vi "Assign Pixel to Wing Sector (FPGA).vi"(4 "End of Data?":bool, 6 "Valid Data?":bool, 7 "Pixel Intensity In":u8, 8 "Right Wing?":bool, 9 "Sector Parameters":T1, 10 "Pixel Y":u16, 11 "Pixel X":u16) -> (0 "Y":u16, 1 "Pixel Intensity Out":u8, 2 "sector #":u8, 3 "output valid":bool, 5 "X":u16)   [LabVIEW 2013]
uses:
  Sector Parameter Cluster.ctl
  <vilib>/rvi/FXPMathLib/FxpRectToPolar/XNode/nifxpmath_RectToPolar.xnode
  <vilib>/rvi/FXPMathLib/FxpSub/XNode/nifxpmath_Sub.xnode
  <vilib>/rvi/FXPMathLib/sim/FxpSim.dll
  <vilib>/rvi/FXPMathLib/FxpAdd/XNode/nifxpmath_Add.xnode
  <vilib>/rvi/FXPMathLib/FxpDiv/XNode/nifxpmath_Div.xnode
  <vilib>/rvi/FXPMathLib/FxpRectToPolar/simVIs/DllFxpRectToPolarTemp_sub.vi
  <vilib>/rvi/FXPMathLib/FxpRectToPolar/subVIs/nifxpmath_RectToPolar_SimConfig.ctl
  <vilib>/ptbypt/NI_PtbyPt.lvlib
  <vilib>/rvi/FXPMathLib/FxpDiv/simVIs/DllFxpDivTemp_sub.vi
  <vilib>/rvi/FXPMathLib/FxpDiv/subVIs/nifxpmath_Div_SimConfig.ctl
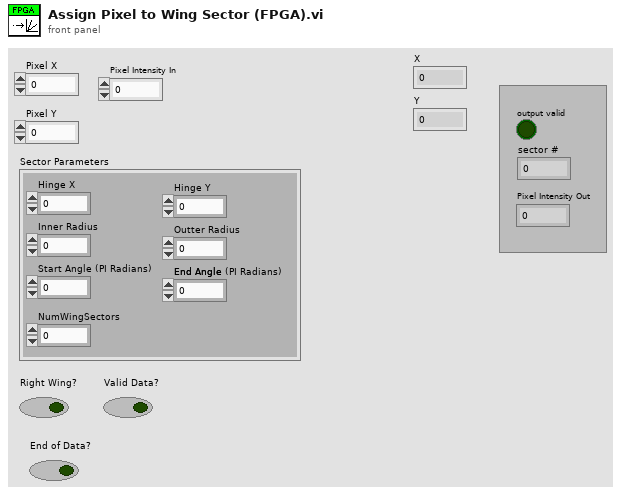
[diagram p1: front panel]
types:
  T1 = typedef "Sector Parameter Cluster.ctl" = cluster{"Start Angle":fxp<+/-,17,2>, "End Angle":fxp<+/-,17,2>, "Inner Radius":u16, "Outter Radius":u16, "Hinge X":u16, "Hinge Y":u16, "NumWingSectors":u8}
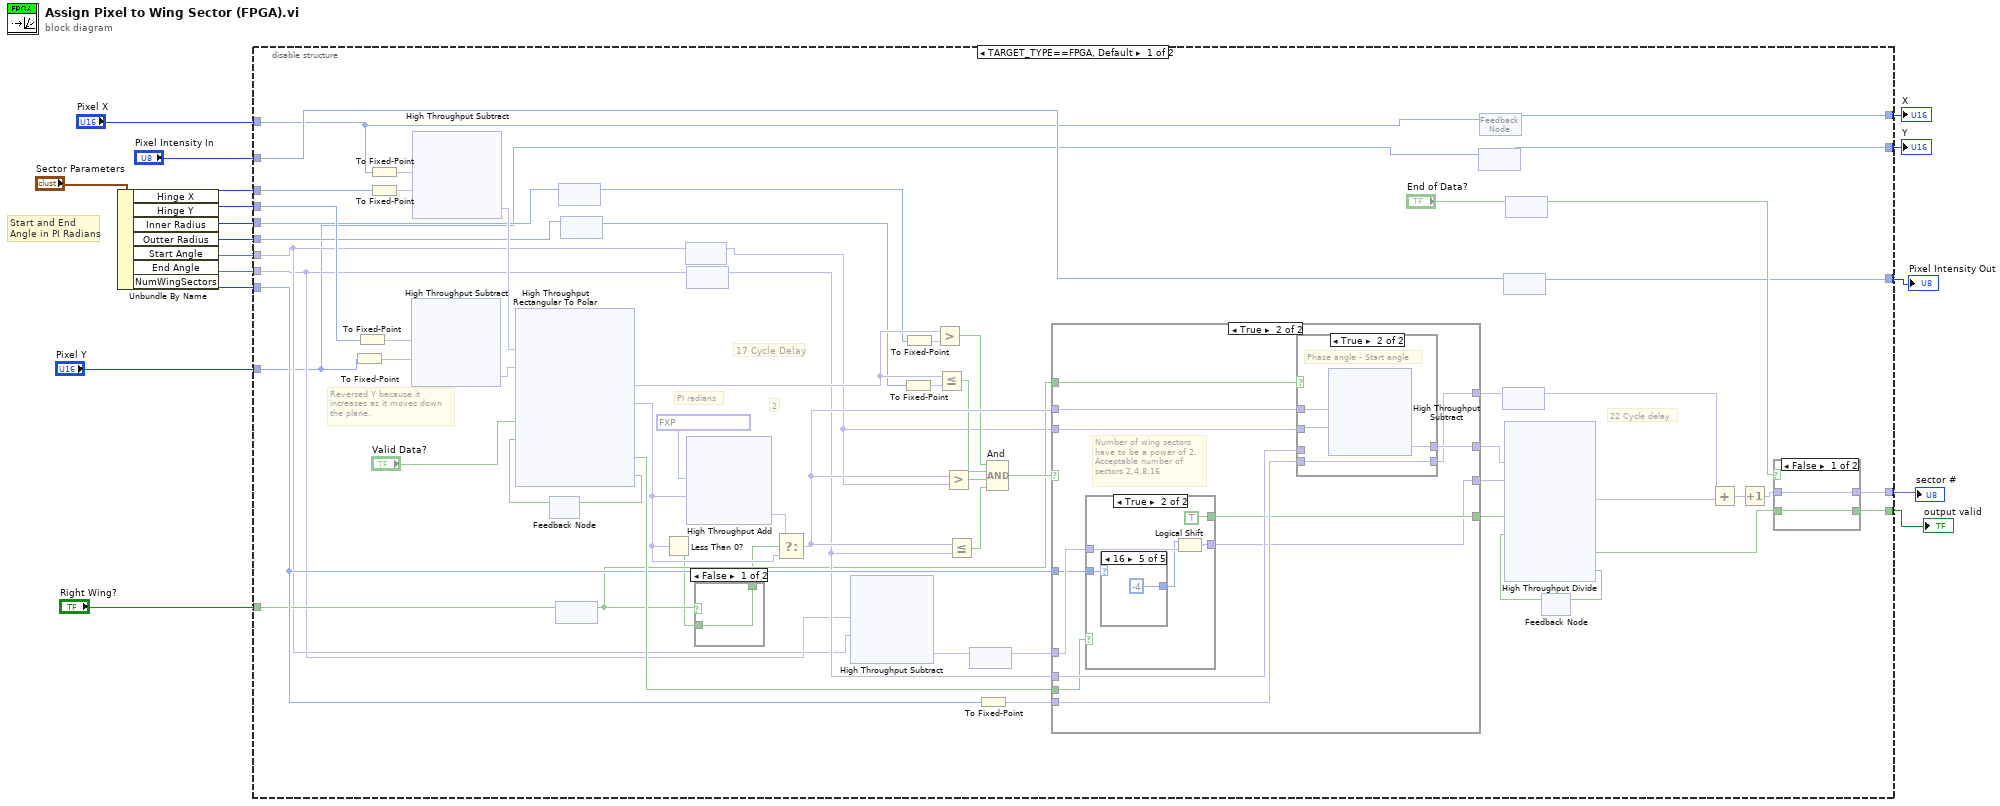
[diagram p0: block diagram]
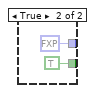
[diagram p2: hidden frame]
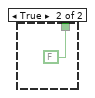
[diagram p3: hidden frame]
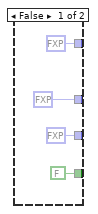
[diagram p4: hidden frame]
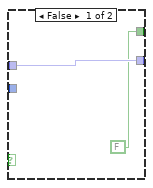
[diagram p5: hidden frame]
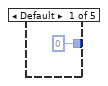
[diagram p6: hidden frame]
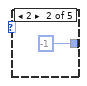
[diagram p7: hidden frame]
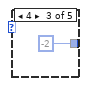
[diagram p8: hidden frame]
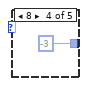
[diagram p9: hidden frame]
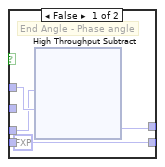
[diagram p10: hidden frame]
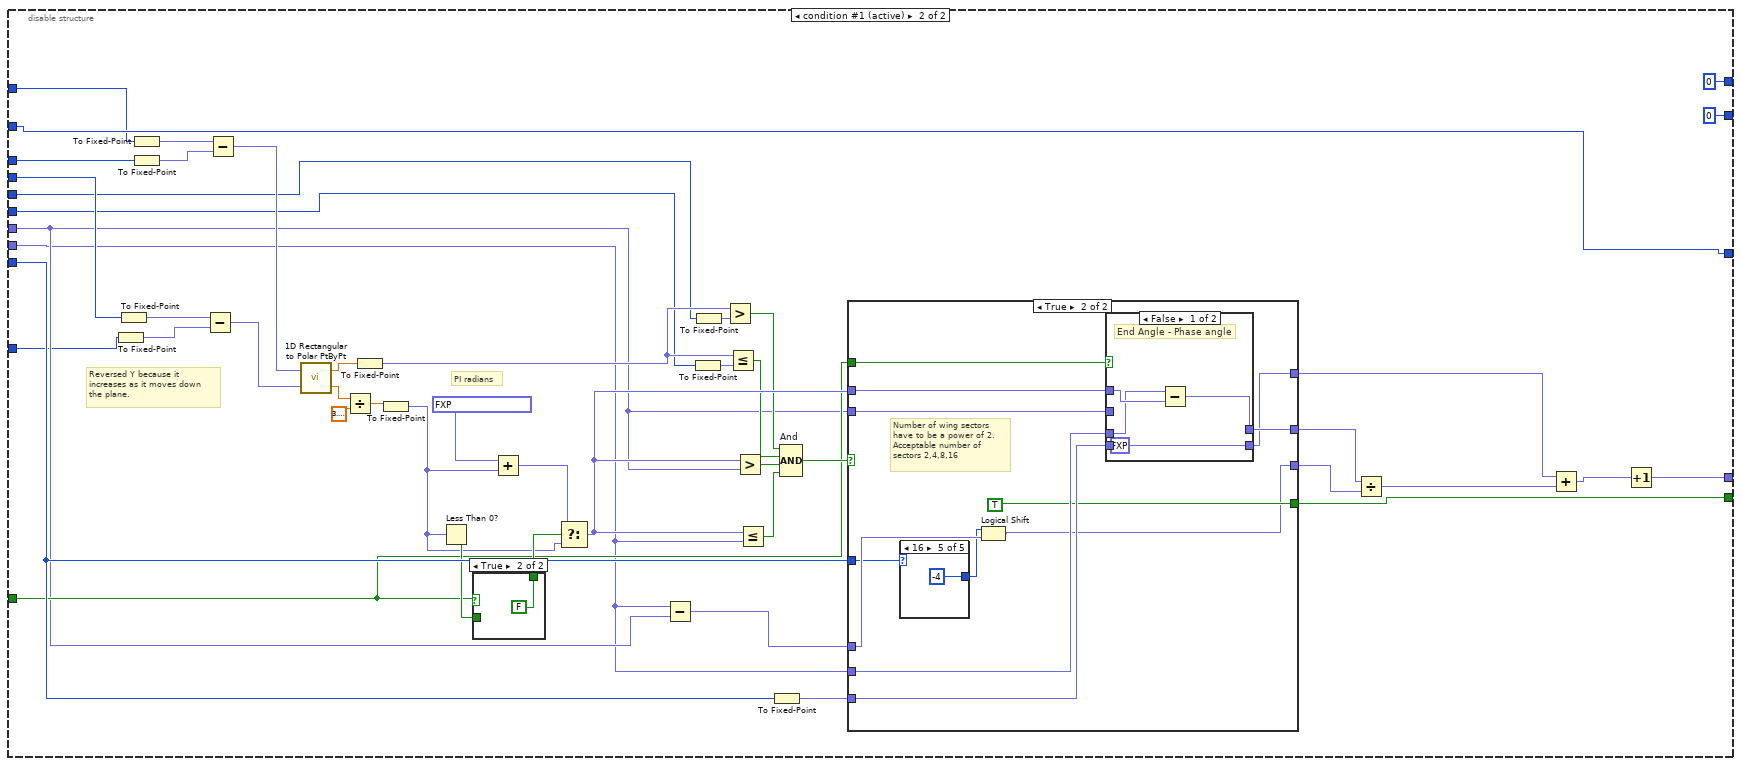
[diagram p11: hidden frame]
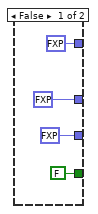
[diagram p13: hidden frame]
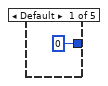
[diagram p14: hidden frame]
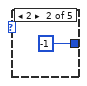
[diagram p15: hidden frame]
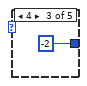
[diagram p16: hidden frame]
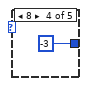
[diagram p17: hidden frame]
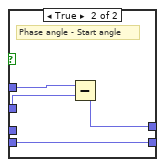
[diagram p18: hidden frame]
diagram:
  # "Start and End\nAngle in PI Radians"
  n1 = Unbundle By Name("Sector Parameters") -> ("Hinge X"=w15:u16, "Hinge Y"=w17:u16, "Inner Radius"=w13:u16, "Outter Radius"=w12:u16, "Start Angle"=w10:fxp<+/-,17,2>, "End Angle"=w9:fxp<+/-,17,2>, "NumWingSectors"=w16:u8)
  n2 = disable-structure shown="TARGET_TYPE==FPGA, Default" {
    disable-tunnel: w17 -> [w64 w224]
    disable-tunnel: w16 -> [w50 w216]
    disable-tunnel: w15 -> [w49 w215]
    disable-tunnel: w13 -> [w48 w204]
    disable-tunnel: w12 -> [w46 w203]
    disable-tunnel: "Right Wing?" -> [w40 w205]
    disable-tunnel: w10 -> [w37 w202]
    disable-tunnel: w9 -> [w35 w201]
    disable-tunnel: [w29 w192] -> w8
    disable-tunnel: [w27 w196] -> w7
    disable-tunnel: "Pixel X" -> [w21 w198]
    disable-tunnel: "Pixel Y" -> [w19 w197]
    disable-tunnel: [w25 w199] -> w4
    disable-tunnel: "Pixel Intensity In" -> [w22 w199]
    disable-tunnel: [w20 u16 0 ("Pixel X")] -> w2
    disable-tunnel: [w18 u16 0 ("Pixel Y")] -> w1
    frame condition #0 {
      # "17 Cycle Delay"
      # "Reversed Y because it\nincreases as it moves down\nthe plane."
      # "PI radians"
      # "22 Cycle delay"
      # "2"
      n3 = To Fixed-Point(number=w19) -> (fixed-point=w54:fxp<+,11,11>)  [unwired: 1 in]
      n4 = To Fixed-Point(number=w64) -> (fixed-point=w55:fxp<+,11,11>)  [unwired: 1 in]
      n5 = To Fixed-Point(number=w21) -> (fixed-point=w53:fxp<+,11,11>)  [unwired: 1 in]
      n6 = To Fixed-Point(number=w49) -> (fixed-point=w52:fxp<+,11,11>)  [unwired: 1 in]
      n7 = xnode "High Throughput Subtract"("x"=w55, "y"=w54) -> ("x-y"=w63:fxp<+/-,12,12>)
      n8 = xnode "High Throughput Subtract"("x"=w53, "y"=w52) -> ("x-y"=w62:fxp<+/-,12,12>)
      n9 = feedback #1() -> (w69:bool)  [unwired: 1 in]
      n10 = xnode "High Throughput Rectangular To Polar"("x"=w62, "y"=w63, "input valid"="Valid Data?", "ready for output (T)"=w69) -> ("magnitude"=w77:fxp<+,12,12>, "phase (pi)"=w74:fxp<+/-,16,2>, "output valid"=w51:bool, "ready for input"=w70:bool)
      n11 = feedback-in #1(w70) -> ()
      n12 = feedback #2() -> (w43:bool)  [unwired: 1 in]
      n13 = feedback-in #2(w40) -> ()
      n14 = feedback #3() -> (w47:u16)  [unwired: 1 in]
      n15 = feedback-in #3(w48) -> ()
      n16 = feedback #4() -> (w45:u16)  [unwired: 1 in]
      n17 = feedback-in #4(w46) -> ()
      n18 = Less Than 0?(x=w74) -> (x < 0?=w41:bool)
      n19 = feedback #5() -> (w36:fxp<+/-,17,2>)  [unwired: 1 in]
      n20 = feedback-in #5(w37) -> ()
      n21 = xnode ("High Throughput Add")("x"=fxp<+/-,16,2> 1.99993896484375 ("y"), "y"=w74) -> ("x+y"=w73:fxp<+/-,17,3>)
      n22 = feedback #6() -> (w44:fxp<+/-,17,2>)  [unwired: 1 in]
      n23 = feedback-in #6(w35) -> ()
      n24 = case shown="False" w43 {
        tunnel: [w83 FALSE ("s")] -> w42
        tunnel: w41 -> [w83 _]
        frame False {
        }
        frame True {
        }
      }
      n25 = Select(t=w73, s=w42, f=w74) -> (s? t:f=w71:fxp<+/-,17,3>)
      n26 = xnode ("High Throughput Subtract")("x"=w35, "y"=w37) -> ("x-y"=w34:fxp<+/-,18,3>)
      n27 = To Fixed-Point(number=w45) -> (fixed-point=w76:fxp<+,16,16>)  [unwired: 1 in]
      n28 = To Fixed-Point(number=w47) -> (fixed-point=w78:fxp<+,16,16>)  [unwired: 1 in]
      n29 = Greater?(x=w77, y=w78) -> (0:w68:bool)
      n30 = Less Or Equal?(x=w77, y=w76) -> (x <= y?=w67:bool)
      n31 = Greater?(x=w71, y=w36) -> (0:w66:bool)
      n32 = Less Or Equal?(x=w71, y=w44) -> (x <= y?=w65:bool)
      n33 = feedback #7() -> (w33:fxp<+/-,18,3>)  [unwired: 1 in]
      n34 = feedback-in #7(w34) -> ()
      n35 = To Fixed-Point(number=w50) -> (fixed-point=w39:fxp<+,8,8>)  [unwired: 1 in]
      n36 = Compound Arithmetic op=AND "And"(w68, w67, w66, w65) -> (w75:bool)
      n37 = case shown="True" w75 {
        tunnel: w71 -> [_ w129]
        tunnel: w36 -> [_ w128]
        tunnel: [fxp<+/-,18,3> 0.0 ("x-y") w119] -> w59
        tunnel: w44 -> [_ w126]
        tunnel: w39 -> [_ w127]
        tunnel: [fxp<+/-,20,5> 0.0 ("x-y") w125] -> w60
        tunnel: [FALSE ("output valid") w120] -> w58
        tunnel: [fxp<+,8,8> 0.0 w124] -> w56
        tunnel: w33 -> [_ w123]
        tunnel: w51 -> [_ w122]
        tunnel: w50 -> [_ w121]
        tunnel: w43 -> [_ w118]
        frame False {
        }
        frame True {
          # "Number of wing sectors\nhave to be a power of 2.\nAcceptable number of\nsectors 2,4,8,16"
          n38 = case shown="True" w122 {
            tunnel: w121 -> [_ w136]
            tunnel: w123 -> [w131 w135]
            tunnel: [w131 w133] -> w119
            tunnel: [FALSE ("output valid") TRUE ("output valid")] -> w120
            frame False {
            }
            frame True {
              n39 = case shown="16" w136 {
                tunnel: [i16 0 ("y") i16 -1 ("y") i16 -2 ("y") i16 -3 ("y") i16 -4 ("y")] -> w134
                frame Default {
                }
                frame 2 {
                }
                frame 4 {
                }
                frame 8 {
                }
                frame 16 {
                }
              }
              n40 = Logical Shift(y=w134, x=w135) -> (x << y=w133:fxp<+/-,18,3>)
            }
          }
          n41 = case shown="True" w118 {
            tunnel: w129 -> [w144 w149]
            tunnel: w128 -> [_ w148]
            tunnel: [w145 w147] -> w125
            tunnel: w127 -> [_ w146]
            tunnel: [fxp<+,8,8> 0.0 w146] -> w124
            tunnel: w126 -> [w143 _]
            frame False {
              # "End Angle - Phase angle"
              n42 = xnode "High Throughput Subtract"("x"=w143, "y"=w144) -> ("x-y"=w145:fxp<+/-,19,4>)
            }
            frame True {
              # "Phase angle - Start angle"
              n43 = xnode ("High Throughput Subtract")("x"=w149, "y"=w148) -> ("x-y"=w147:fxp<+/-,19,4>)
            }
          }
        }
      }
      n44 = feedback #8() -> (w18:u16)  [unwired: 1 in]
      n45 = feedback-in #8(w19) -> ()
      n46 = feedback-in #9(w21) -> ()
      n47 = feedback #9() -> (w20:u16)  [unwired: 1 in]
      n48 = feedback #10() -> (w38:fxp<+,8,8>)  [unwired: 1 in]
      n49 = feedback-in #10(w56) -> ()
      n50 = feedback #11() -> (w25:u8)  [unwired: 1 in]
      n51 = feedback-in #11(w22) -> ()
      n52 = feedback #12() -> (w30:bool)  [unwired: 1 in]
      n53 = feedback-in #12("End of Data?") -> ()
      n54 = feedback #13() -> (w57:bool)  [unwired: 1 in]
      n55 = xnode "High Throughput Divide"("x"=w60, "y"=w59, "input valid"=w58, "ready for output (T)"=w57) -> ("x/y"=w24:fxp<+/-,20,20>, "output valid"=w26:bool, "ready for input"=w61:bool)
      n56 = feedback-in #13(w61) -> ()
      n57 = Add(x=w38, y=w24) -> (x+y=w28:fxp<+/-,21,21>)
      n58 = Increment(x=w28) -> (x+1=w23:fxp<+/-,21,21>)
      n59 = case shown="False" w30 {
        tunnel: [w80 fxp<+/-,17,17> 0.0] -> w29
        tunnel: w23 -> [w80 _]
        tunnel: [w79 TRUE ("output valid")] -> w27
        tunnel: w26 -> [w79 _]
        frame False {
        }
        frame True {
        }
      }
    }
    frame condition #1 (active) {
      # "Reversed Y because it\nincreases as it moves down\nthe plane."
      # "PI radians"
      n60 = To Fixed-Point(number=w197) -> (fixed-point=w219:fxp<+,11,11>)  [unwired: 1 in]
      n61 = To Fixed-Point(number=w224) -> (fixed-point=w220:fxp<+,11,11>)  [unwired: 1 in]
      n62 = To Fixed-Point(number=w198) -> (fixed-point=w218:fxp<+,11,11>)  [unwired: 1 in]
      n63 = To Fixed-Point(number=w215) -> (fixed-point=w217:fxp<+,11,11>)  [unwired: 1 in]
      n64 = Subtract(x=w220, y=w219) -> (x-y=w223:fxp<+/-,12,12>)
      n65 = Subtract(x=w218, y=w217) -> (x-y=w222:fxp<+/-,12,12>)
      n66 = call <vilib>:"1D Rectangular to Polar PtByPt.vi"("y"=w223, "x"=w222) -> ("phase"=w209:dbl, "magnitude"=w211:dbl)
      n67 = Divide(x=w209, y=3.141592653589793) -> (x/y=w207:dbl)
      n68 = To Fixed-Point(number=w211) -> (fixed-point=w210:fxp<+,12,12>)  [unwired: 1 in]
      n69 = To Fixed-Point(number=w207) -> (fixed-point=w206:fxp<+/-,16,2>)  [unwired: 1 in]
      n70 = Less Than 0?(x=w206) -> (x < 0?=w213:bool)
      n71 = case shown="True" w205 {
        tunnel: [w235 FALSE ("s")] -> w214
        tunnel: w213 -> [w235 _]
        frame False {
        }
        frame True {
        }
      }
      n72 = Add(x=fxp<+/-,16,2> 1.99993896484375 ("y"), y=w206) -> (x+y=w231:fxp<+/-,17,3>)
      n73 = Select(t=w231, s=w214, f=w206) -> (s? t:f=w229:fxp<+/-,17,3>)
      n74 = Subtract(x=w201, y=w202) -> (x-y=w200:fxp<+/-,18,3>)
      n75 = To Fixed-Point(number=w203) -> (fixed-point=w233:fxp<+,16,16>)  [unwired: 1 in]
      n76 = To Fixed-Point(number=w204) -> (fixed-point=w234:fxp<+,16,16>)  [unwired: 1 in]
      n77 = Greater?(x=w210, y=w234) -> (0:w228:bool)
      n78 = Less Or Equal?(x=w210, y=w233) -> (x <= y?=w227:bool)
      n79 = Greater?(x=w229, y=w202) -> (0:w226:bool)
      n80 = Less Or Equal?(x=w229, y=w201) -> (x <= y?=w225:bool)
      n81 = To Fixed-Point(number=w216) -> (fixed-point=w212:fxp<+,8,8>)  [unwired: 1 in]
      n82 = Compound Arithmetic op=AND "And"(w228, w227, w226, w225) -> (w232:bool)
      n83 = case shown="True" w232 {
        tunnel: w229 -> [_ w252]
        tunnel: w202 -> [_ w251]
        tunnel: [fxp<+/-,18,3> 0.0 ("x-y") w243] -> w194
        tunnel: w201 -> [_ w249]
        tunnel: w212 -> [_ w250]
        tunnel: [fxp<+/-,20,5> 0.0 ("x-y") w248] -> w221
        tunnel: [FALSE ("output valid") TRUE ("output valid")] -> w196
        tunnel: [fxp<+,8,8> 0.0 w247] -> w195
        tunnel: w200 -> [_ w246]
        tunnel: w216 -> [_ w245]
        tunnel: w205 -> [_ w242]
        frame False {
        }
        frame True {
          # "Number of wing sectors\nhave to be a power of 2.\nAcceptable number of\nsectors 2,4,8,16"
          n84 = case shown="16" w245 {
            tunnel: [i16 0 ("y") i16 -1 ("y") i16 -2 ("y") i16 -3 ("y") i16 -4 ("y")] -> w241
            frame Default {
            }
            frame 2 {
            }
            frame 4 {
            }
            frame 8 {
            }
            frame 16 {
            }
          }
          n85 = Logical Shift(y=w241, x=w246) -> (x << y=w243:fxp<+/-,18,3>)
          n86 = case shown="False" w242 {
            tunnel: w252 -> [w260 w265]
            tunnel: w251 -> [_ w264]
            tunnel: [w261 w263] -> w248
            tunnel: w250 -> [_ w262]
            tunnel: [fxp<+,8,8> 0.0 w262] -> w247
            tunnel: w249 -> [w259 _]
            frame False {
              # "End Angle - Phase angle"
              n87 = Subtract(x=w259, y=w260) -> (x-y=w261:fxp<+/-,19,4>)
            }
            frame True {
              # "Phase angle - Start angle"
              n88 = Subtract(x=w265, y=w264) -> (x-y=w263:fxp<+/-,19,4>)
            }
          }
        }
      }
      n89 = Divide(x=w221, y=w194) -> (x/y=w191:fxp<+/-,20,20>)
      n90 = Add(x=w195, y=w191) -> (x+y=w193:fxp<+/-,21,21>)
      n91 = Increment(x=w193) -> (x+1=w192:fxp<+/-,21,21>)
    }
  }
  "output valid" <- w7
  "sector #" <- w8
  "Pixel Intensity Out" <- w4
  "X" <- w2
  "Y" <- w1
